vi "inst.JIG_TRIGGER.vi"(7 "unit ID (1)":u8=1, 8 "error in (no error)":errorcluster, 11 "Modbus master in":refnum<class "Modbus Master.lvclass">) -> (0 "error out":errorcluster, 1 "INPUT0":bool, 2 "JIG_TRIGGER":bool, 3 "Modbus master out":refnum<class "Modbus Master.lvclass">)   [LabVIEW 2018, in "MB Relay.lvlib"]
uses:
  MB Relay.lvlib
  <vilib>/NI/Modbus Library/API/Master/Modbus Master.lvclass
  type defs/MB relays _InstrumentType.ctl
  type defs/FGV enum.ctl
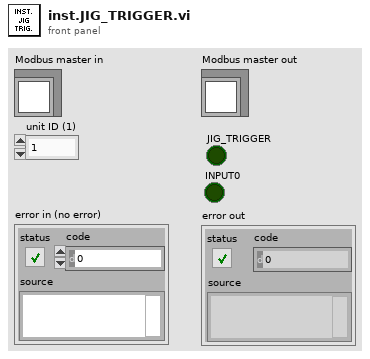
[diagram p1: front panel]
types:
  T1 = typedef "MB Relay.lvlib/FGV enum.ctl" = enum16{"Write", "Init FGV", "Read", "All OFF", "All ON"}
  T2 = typedef "MB Relay.lvlib/MB relays _InstrumentType.ctl" = enum16{"JIG_TRIGGER", "JIG_RESET", "Relay SelfTest", "counter", "demux1_10(x6)", "mux10_1(x6)", "mux6_1(3wires)", "MB_Relay_01(eMICs)", "SpareRelays(DPDT)", "Optos", "Inputs", "DMM I 0.5", "SpareRelays (SPDT)", "SC enable"}
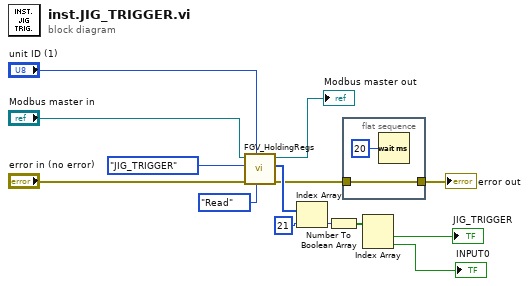
[diagram p0: block diagram]
diagram:
  n1 = call "FGV_HoldingRegs.vi"("FGV_enum"=FGV_enum."Read", "unit ID"="unit ID (1)", "error in (no error)"="error in (no error)", "Instruments"=MB_relays__InstrumentType."JIG_TRIGGER", "Modbus master in"="Modbus master in") -> ("error out"=w1:errorcluster, "HoldingRegs"=w9:u16[], "Modbus master out"=→"Modbus master out":refnum<class "Modbus Master.lvclass">)  [unwired: 4 in]
  n2 = Index Array(array=w9, index=21) -> (element=w7:u16)
  n3 = Number To Boolean Array(number=w7) -> (Boolean array=w6:bool[])
  n4 = flat-sequence {
    tunnel: [w15] -> w2
    tunnel: w1 -> [w15]
    frame #0 {
      n5 = Wait (ms)(milliseconds to wait=u32 20) -> ()  [unwired: 1 out]
    }
  }
  n6 = Index Array(array=w6) -> (element #1=→"JIG_TRIGGER":bool, element #2=→"INPUT0":bool)  [unwired: 2 in]
  "error out" <- w2
